vi "DMSV.close_info_panels.vi"(0 "infoPanels":refnum<vi>[](array[refnum]), 2 "panel@node":string[](array[string]), 5 "error in (no error)":errorcluster) -> (14 "infoPanels out":refnum<vi>[](array[refnum]), 16 "panel@node out":string[](array[string]), 19 "error out":errorcluster)   [LabVIEW 2014, in "DMSViewer.lvlib"]
doc: "Checks if the infoPanels are closed. If yes, then destroy panel.\n\nauthor: Dietrich Beck, GSI\n\nLicense Agreement for this software:\n\nCopyright (C)\nGesellschaft für Schwerionenforschung, GSI\nPlanckstr. 1\n64291 Darmstadt\nGermany\n\nContact: D.Beck@gsi.de \n\nThis program is free software; you can redistribute it and/or modify it under the terms of the GNU General Public License as published by the Free Software Foundation; either version 2 of the license, or (at your option) any later version.\n\nThis program is distributed in the hope that it will be useful, but WITHOUT ANY WARRANTY; without even the implied warranty of MERCHANTABILITY or FITNESS FOR A PARTICULAR PURPOSE. See the GNU General License for more details (http://www.gnu.org).\n\nGesellschaft für Schwerionenforschung, GSI\nPlanckstr. 1, 64291 Darmstadt, Germany\nFor all questions and ideas contact: M.Richter@gsi.de, H.Brand@gsi.de or D.Beck@gsi.de.\nLast update: 10-OCT-2004"
uses:
  DMSViewer.lvlib
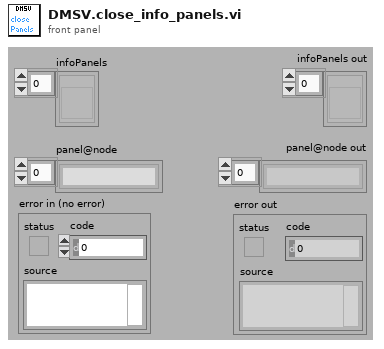
[diagram p1: front panel]
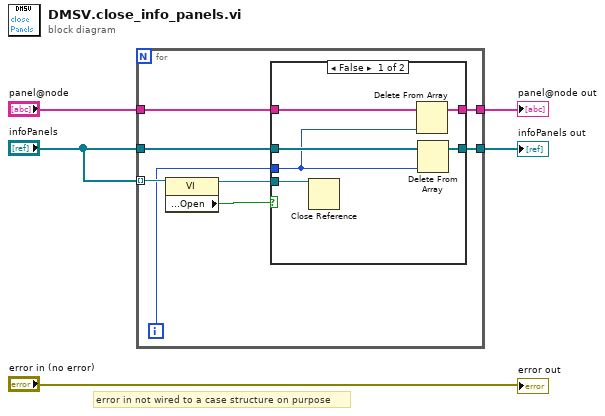
[diagram p0: block diagram]
diagram:
  # "error in not wired to a case structure on purpose"
  n1 = for {
    tunnel: "infoPanels" -> [w12] mode=indexing
    tunnel: "infoPanels" -> [w13]
    tunnel: [w8] -> w4
    tunnel: "panel@node" -> [w7]
    tunnel: [w6] -> w1
    i -> [w9]
    n2 = property on="Property Node" class="VI"(reference=w12) -> (reference out=w10:refnum<vi>, "Front Panel Window:Open"=w11:bool)  [unwired: 1 in, 1 out]
    n3 = case shown="False" w11 {
      tunnel: w13 -> [w19 w21]
      tunnel: w10 -> [w18 _]
      tunnel: w9 -> [w15 _]
      tunnel: [w17 w21] -> w8
      tunnel: w7 -> [w16 w20]
      tunnel: [w14 w20] -> w6
      frame False {
        n4 = Close Reference(reference=w18) -> ()  [unwired: 1 in, 1 out]
        n5 = Delete From Array(array=w16, index=w15) -> (array with subset deleted=w14:string[])  [unwired: 1 in, 1 out]
        n6 = Delete From Array(array=w19, index=w15) -> (array with subset deleted=w17:refnum<vi>[])  [unwired: 1 in, 1 out]
      }
      frame True {
      }
    }
  }
  "infoPanels out" <- w4
  "panel@node out" <- w1
  "error out" <- "error in (no error)"
